vi "Error (SubVI).vi"(8 "error in (no error)":errorcluster, 11 "VISA Refnum in":refnum<visa-resource-name>) -> (0 "error out":errorcluster, 1 "Error Message":string, 2 "Error Code":i32[](array[numeric]), 3 "VISA Refnum out":refnum<visa-resource-name>)   [LabVIEW 2023]
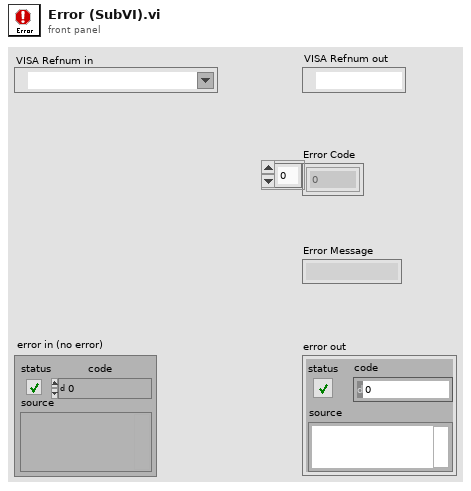
[diagram p1: front panel]
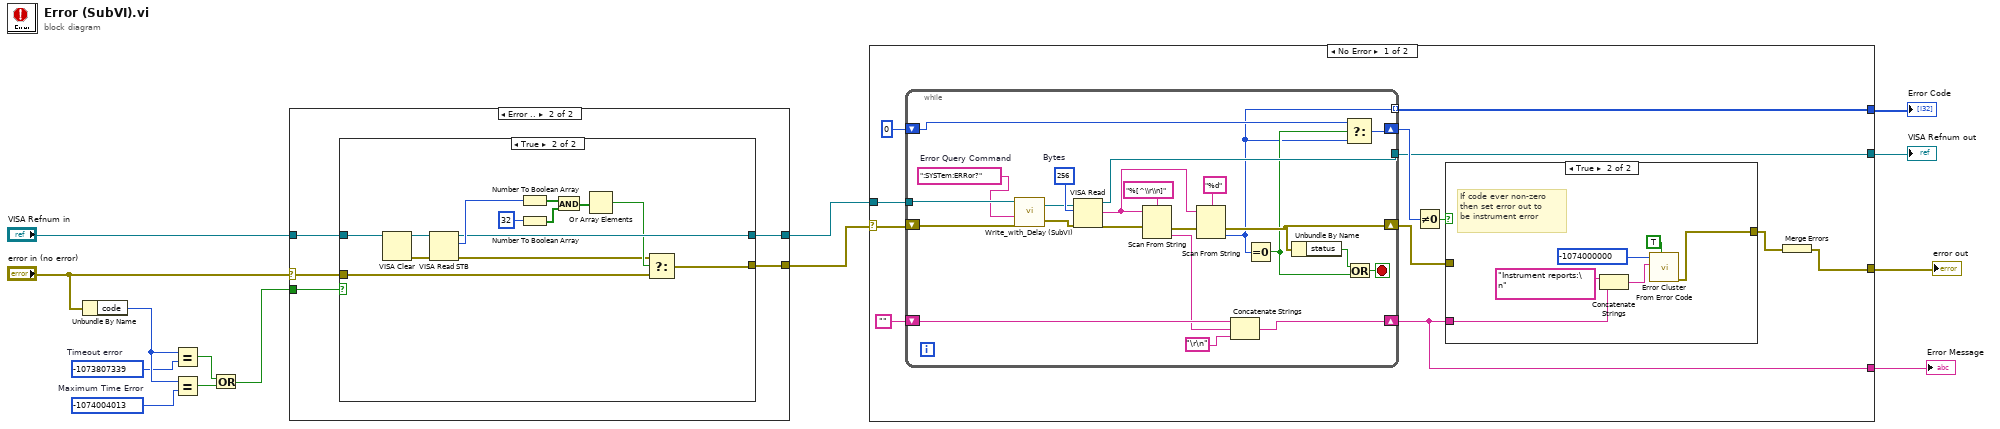
[diagram p0: block diagram]
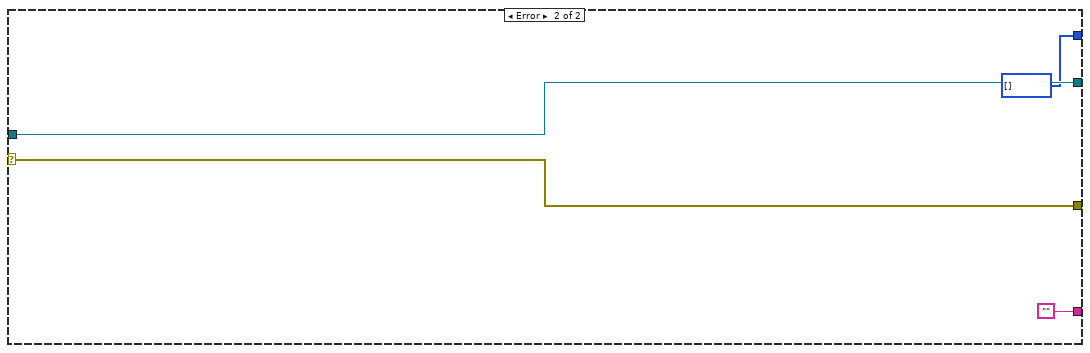
[diagram p3: hidden frame]
diagram:
  w4 = -1074004013  # Maximum Time Error
  w3 = -1073807339  # Timeout error
  n1 = Unbundle By Name("error in (no error)") -> ("code"=w7:i32)
  n2 = Equal?(x=w7, y=w3) -> (x = y?=w6:bool)
  n3 = Equal?(x=w7, y=w4) -> (x = y?=w5:bool)
  n4 = Or(x=w6, y=w5) -> (x .or. y?=w8:bool)
  n5 = case shown="Error .." "error in (no error)" {
    selector: "error in (no error)" -> [w15 w19]
    tunnel: "VISA Refnum in" -> [w16 w20]
    tunnel: w8 -> [_ w21]
    tunnel: [w16 w18] -> w10
    tunnel: [w15 w17] -> w9
    frame No Error {
    }
    frame Error {
      n6 = case shown="True" w21 {
        tunnel: w20 -> [w23 w36]
        tunnel: w19 -> [w22 w25]
        tunnel: [w23 w28] -> w18
        tunnel: [w22 w24] -> w17
        frame False {
        }
        frame True {
          n7 = VISA Clear(VISA resource name=w36) -> (VISA resource name out=w34:refnum<visa-resource-name>, error out=w35:errorcluster)  [unwired: 1 in]
          n8 = VISA Read STB(8:w35, 11:w34) -> (0:w26:errorcluster, 2:w29:u16, 3:w28:refnum<visa-resource-name>)
          n9 = Number To Boolean Array(number=w29) -> (Boolean array=w30:bool[])
          n10 = Number To Boolean Array(number=32) -> (Boolean array=w32:bool[])
          n11 = And(x=w30, y=w32) -> (x .and. y?=w31:bool[])
          n12 = Or Array Elements(Boolean array=w31) -> (logical OR=w27:bool)
          n13 = Select(t=w26, s=w27, f=w25) -> (s? t:f=w24:errorcluster)
        }
      }
    }
  }
  n14 = case shown="No Error" w9 {
    selector: w9 -> [w42 w81]
    tunnel: w10 -> [w43 w82]
    tunnel: [w40 w82] -> w12
    tunnel: [w37 w81] -> w13
    tunnel: [w39 i32[] []] -> w11
    tunnel: [w41 ""] -> w14
    frame No Error {
      n15 = while {
        tunnel: [w78] -> w40
        tunnel: w43 -> [w60]
        shift-right: [w69] -> w41
        shift-left: "" -> [w72]
        shift-right: [w67] -> w45
        shift-left: 0 -> [w68]
        shift-right: [w66] -> w44
        shift-left: w42 -> [w59]
        tunnel: [w61] -> w39 mode=indexing
        stop <- w75 stop-if-true
        w77 = u32 256  # Bytes
        w58 = ":SYSTem:ERRor?"  # Error Query Command
        n16 = call "Write_with_Delay (SubVI).vi"("error in (no error)"=w59, "Command"=w58, "VISA Refnum in"=w60) -> ("error out"=w56:errorcluster, "VISA Refnum out"=w57:refnum<visa-resource-name>)  [unwired: 1 in]
        n17 = VISA Read(VISA resource name=w57, byte count=w77, error in (no error)=w56) -> (VISA resource name out=w78:refnum<visa-resource-name>, read buffer=w73:string, error out=w65:errorcluster)  [unwired: 1 out]
        n18 = Scan From String(format string="%[^\\r\\n]", input string=w73, error in=w65) -> (error out=w64:errorcluster, output 1=w70:string)  [unwired: 1 in, 3 out]
        n19 = Scan From String(format string="%d", input string=w73, error in=w64) -> (error out=w66:errorcluster, output 1=w61:i32)  [unwired: 1 in, 3 out]
        n20 = Concatenate Strings(w72, w70, "\r\n") -> (w69:string)
        n21 = Equal To 0?(x=w61) -> (x = 0?=w62:bool)
        n22 = Unbundle By Name(w66) -> ("status"=w63:bool)
        n23 = Select(t=w68, s=w62, f=w61) -> (s? t:f=w67:i32)
        n24 = Or(x=w63, y=w62) -> (x .or. y?=w75:bool)
      }
      n25 = Not Equal To 0?(x=w45) -> (x != 0?=w46:bool)
      n26 = case shown="True" w46 {
        tunnel: w41 -> [_ w54]
        tunnel: [w49 w50] -> w38
        tunnel: w44 -> [w49 _]
        frame False {
        }
        frame True {
          # "If code ever non-zero\nthen set error out to\nbe instrument error"
          n27 = Concatenate Strings("Instrument reports:\n" ("Source"), w54) -> (w51:string)
          n28 = call <vilib>:"Error Cluster From Error Code.vi"("show call chain? (False)"=TRUE, "error message (\"\")"=w51, "error code (0)"=-1074000000 ("Code")) -> ("error out"=w50:errorcluster)  [unwired: 1 in, 5 out]
        }
      }
      n29 = Merge Errors(w38) -> (w37:errorcluster)
    }
    frame Error {
    }
  }
  "Error Code" <- w11
  "VISA Refnum out" <- w12
  "error out" <- w13
  "Error Message" <- w14
